vi "Escape Label.vi"(8 "error in (no error)":errorcluster, 11 "Label":string) -> (0 "error out":errorcluster, 3 "YAML Label":string)   [LabVIEW 2015, in "YAML Parser.lvlib"]
uses:
  YAML Parser.lvlib
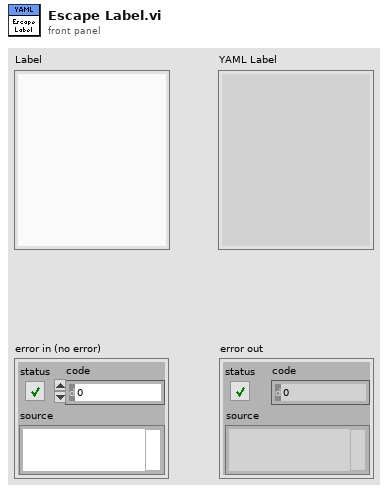
[diagram p1: front panel]
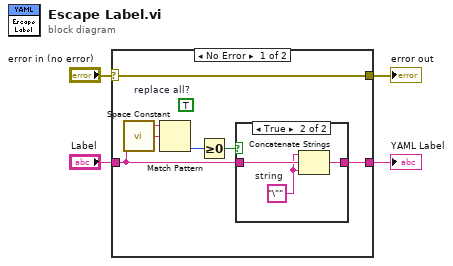
[diagram p0: block diagram]
diagram:
  n1 = case shown="No Error" "error in (no error)" {
    selector: "error in (no error)" -> [w10 w15]
    tunnel: [w10 w15] -> w3
    tunnel: "Label" -> [w5 w16]
    tunnel: [w6 w16] -> w1
    frame No Error {
      (unwired) TRUE  # replace all?
      n2 = call <vilib>:"Space Constant.vi"() -> ("String"=w9:string)
      n3 = Match Pattern(string=w5, regular expression=w9) -> (offset past match=w8:i32)  [unwired: 1 in, 3 out]
      n4 = Greater Or Equal To 0?(x=w8) -> (x >= 0?=w7:bool)
      n5 = case shown="True" w7 {
        tunnel: [w11 w12] -> w6
        tunnel: w5 -> [w11 w14]
        frame False {
        }
        frame True {
          w13 = "\""  # string
          n6 = Concatenate Strings(w13, w14, w13) -> (w12:string)
        }
      }
    }
    frame Error {
    }
  }
  "error out" <- w3
  "YAML Label" <- w1
